vi "R vs T measurement.vi"() -> ()   [LabVIEW 2017]
uses:
  <vilib>/Utility/file.llb/Read Delimited Spreadsheet (DBL).vi
  <vilib>/Utility/file.llb/Write Delimited Spreadsheet (DBL).vi
  <instrlib>/Lake Shore 336/Lake Shore 336.lvlib
panel:
  in  "Tab Control":enum32{"Controlls", "Graphs"}(tab)
  in  "Source Meter address":refnum<visa-resource-name>="GPIB1::29::INSTR"
  out "Measured Resistance (Ohms)":dbl format="%#_6p"
  in  "Resistance Range Lower Limit (2 Ohm)":dbl=2.0 format="%#_6p"
  in  "Resistance Range Upper Limit (2E+8 Ohm)":dbl=200000000.0 format="%#_6p"
  in  "Resistance NPLC (0.1)":dbl=0.1
  in  "Resistance Range (2 Ohm)":dbl=2.0
  in  "Resistance Auto Range (T: Enable)":bool=TRUE
  in  "file to save data (dialog if empty)":path
  in  "Temperature controller Addres":refnum<visa-resource-name>
  in  "Input (0:A)":u16(ring) items=["A", "B", "C", "D"]
  in  "Range (0:Off)":u16(ring) items=["Off", "Low (On)", "Medium", "High"]
  in  "Manual Output (0.00 %)":dbl format="%.2f"
  in  "Setpoint (0.00000)":dbl format="%.5f"
  in  "Enable Setpoint (F:Off)":bool
  out "Measured Resistance (K)":dbl format="%.6p"
  in  "Ramp Rate (0.0)":dbl format="%.1f"
  in  "Setpoint Ramping \nEnable (F: Off)":bool
  in  "Output's Control Loop (1:1)":u16(ring)=1 items=["1"=1, "2"=2]
  in  "Rate (D) (0.0 %)":dbl format="%.1f"
  in  "Reset (I) (20.0)":dbl=20.0 format="%.1f"
  in  "Gain (P) (50.0)":dbl=50.0 format="%.1f"
  in  "Mode (0:Off)":u16(ring) items=["Off", "Closed Loop PID", "Zone", "Open Loop"]
  in  "Max User Current (2.000)":dbl=2.0 format="%.3f"
  in  "Max Current (0:User Specified)":u16(ring) items=["User Specified", "0.707 A", "1.0 A", "1.141 A", "2.0 A"]
  in  "Heater Out Display (1:Current)":u16(ring)=1 items=["Current"=1, "Power"=2]
  in  "Heater Resistance (1:25 Ohms)":u16(ring)=1 items=["25 Ohms"=1, "50 Ohms"=2]
  in  "Record Rate (ms)":u32=1000
  out "R T Graph":cluster{"all rows":dbl[], "all rows":dbl[]}(graph)
  in  "stop":bool
  in  "Error In":errorcluster
  # "Resistance vs Temperature Measurement"
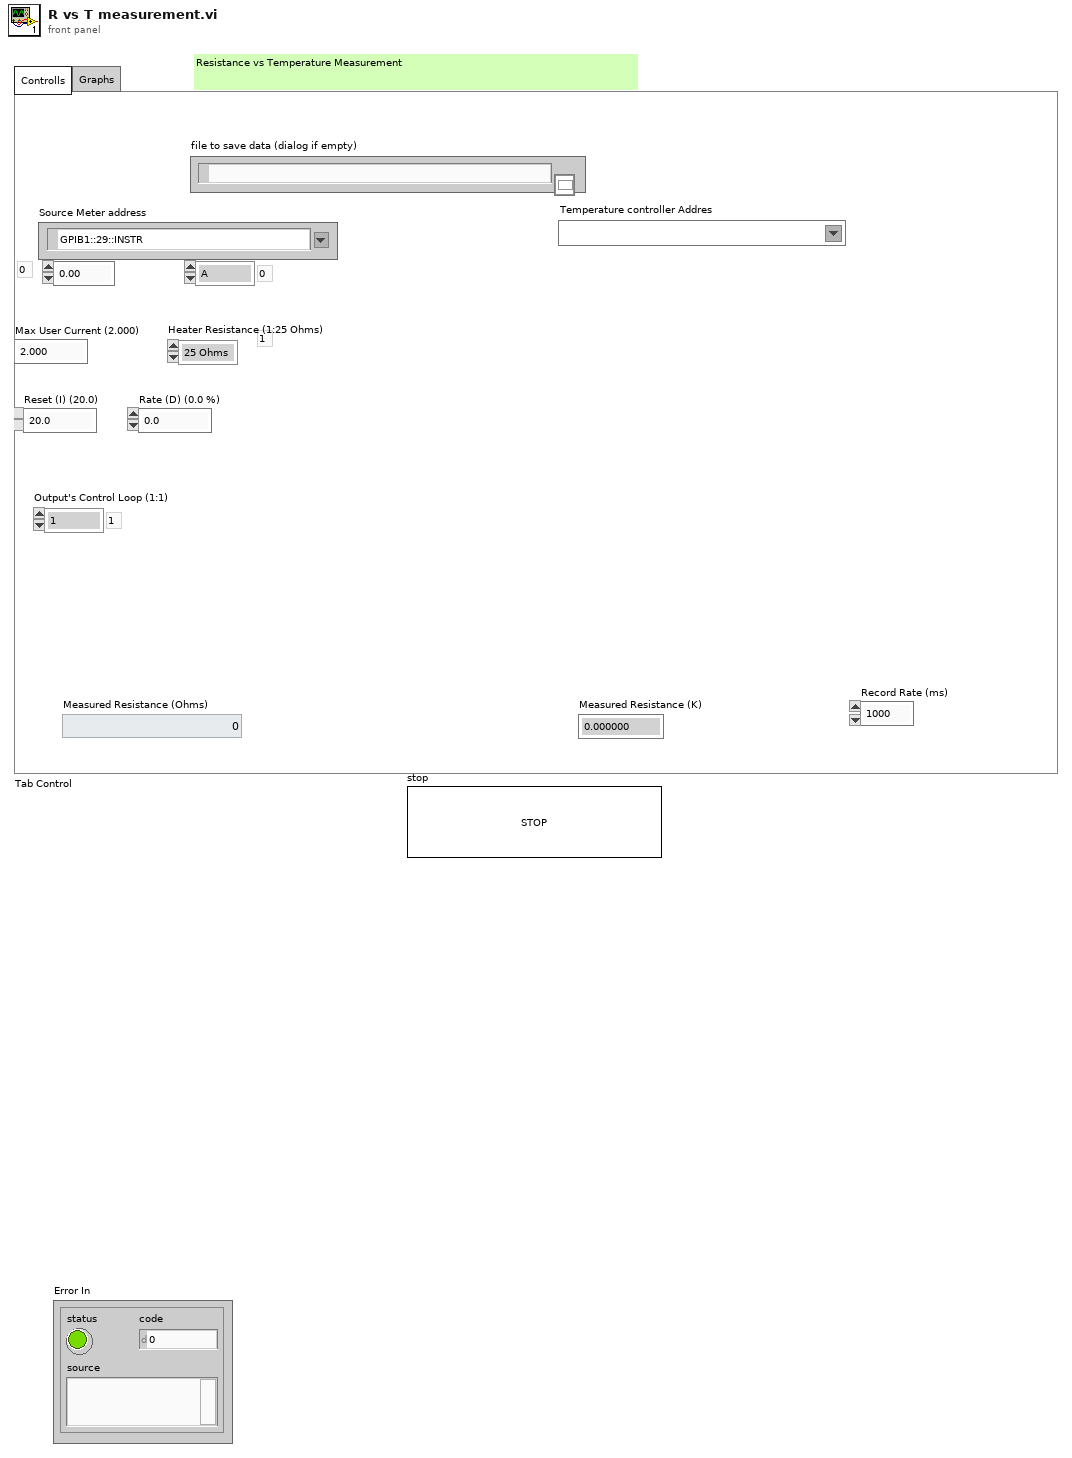
[diagram p1: front panel]
types:
  T1 = cluster{"Baud Rate":u32, "Parity":u16, "Data Bits":u16, "Stop Bits":u16, "Flow Control":u16}
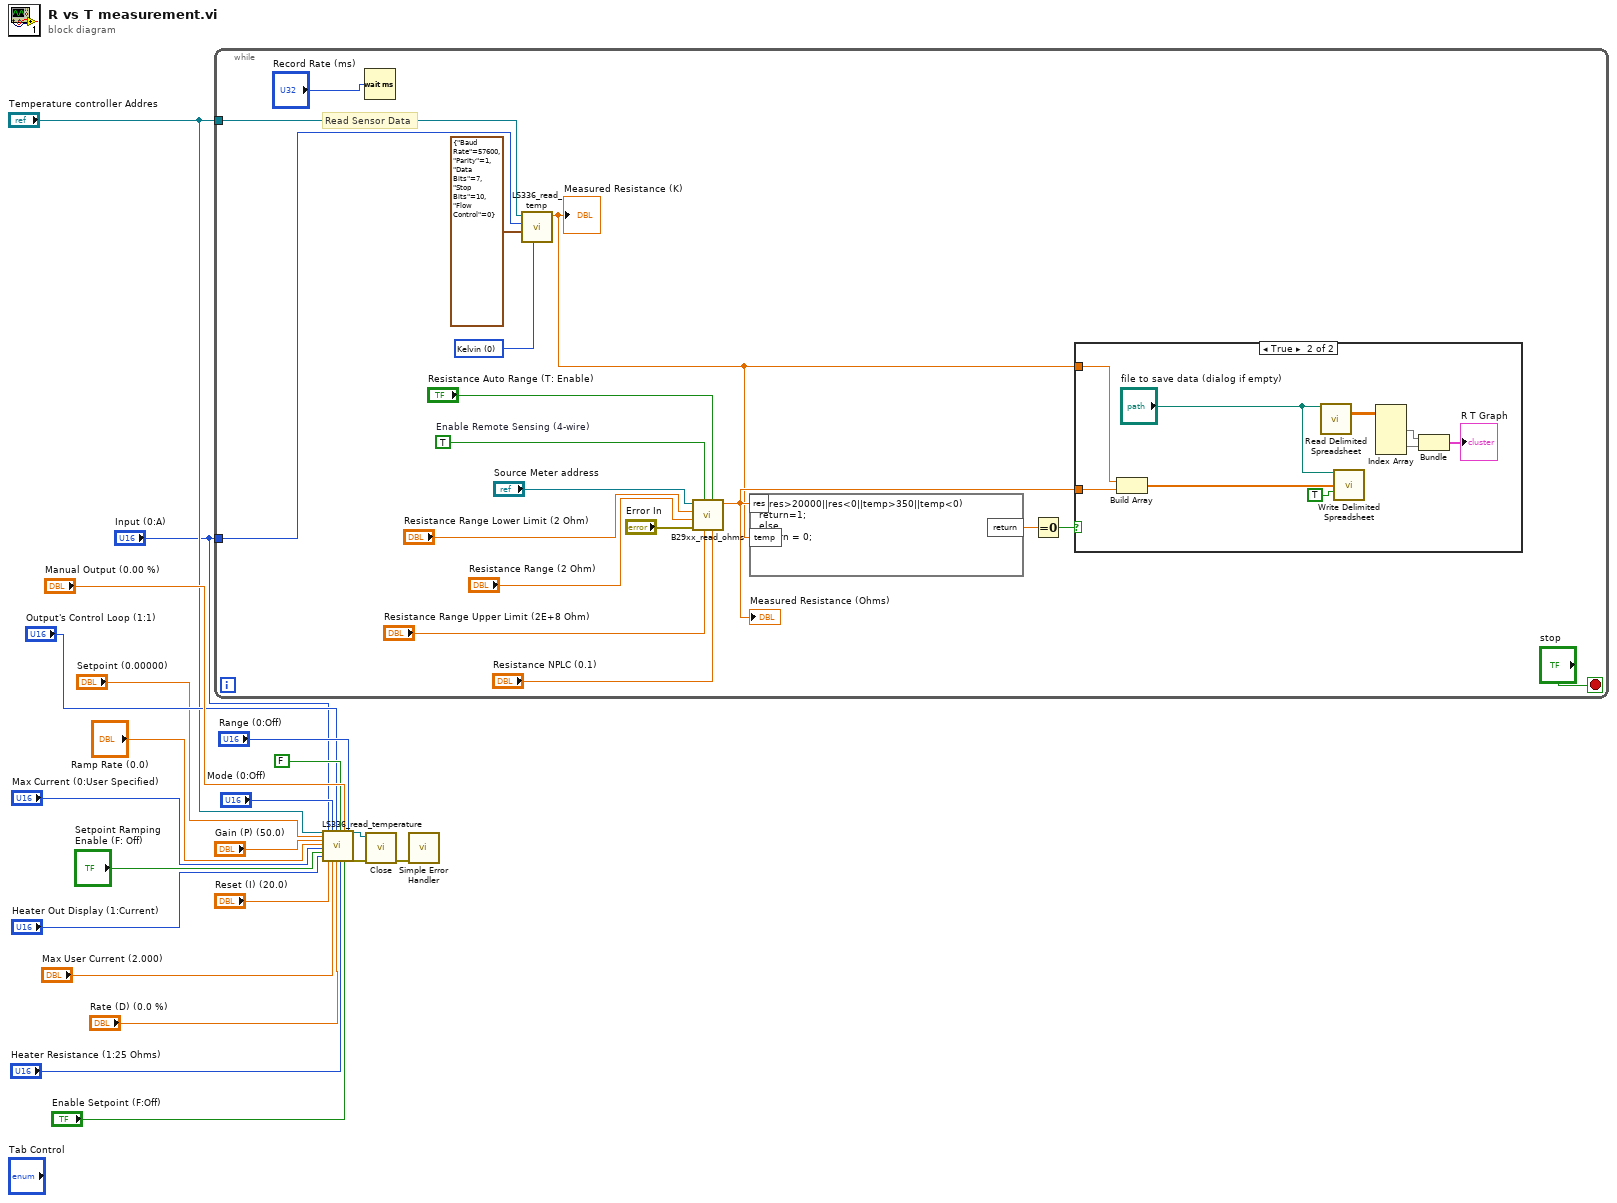
[diagram p0: block diagram]
diagram:
  n1 = while {
    tunnel: "Temperature controller Addres" -> [w23]
    tunnel: "Input (0:A)" -> [w22]
    stop <- "stop" stop-if-true
    w25 = u16 0 items=["Kelvin", "Celsius", "Sensor Units"] ("Data Source (0:Kelvin)")
    w37 = TRUE  # Enable Remote Sensing (4-wire)
    # "Read Sensor Data"
    n2 = Wait (ms)(milliseconds to wait="Record Rate (ms)") -> ()  [unwired: 1 out]
    n3 = call "LS336_read_temp.vi"("Data Source (0:Kelvin)"=w25, "Serial Configuration"=T1 {"Baud Rate"=57600, "Parity"=1, "Data Bits"=7, "Stop Bits"=10, "Flow Control"=0}, "Input (0:A)"=w22, "VISA Refnum in"=w23) -> ("Sensor Data"=w24:dbl)  [unwired: 7 in]
    "Measured Resistance (K)" <- w24
    n4 = call "B29xx_read_ohms.vi"("Resistance NPLC (0.1)"="Resistance NPLC (0.1)", "Resistance Auto Range (T: Enable)"="Resistance Auto Range (T: Enable)", "Resistance Range Upper Limit (2E+8 Ohm)"="Resistance Range Upper Limit (2E+8 Ohm)", "Enable Remote Sensing (4-wire)"=w37, "error in (no error)"="Error In", "Resistance Range (2 Ohm)"="Resistance Range (2 Ohm)", "Resistance Range Lower Limit (2 Ohm)"="Resistance Range Lower Limit (2 Ohm)", "VISA Refnum in"="Source Meter address") -> ("Measurement Result"=w29:dbl)  [unwired: 2 in, 1 out]
    "Measured Resistance (Ohms)" <- w29
    n5 = formula code="if(res>20000||res<0||temp>350||temp<0)\nreturn=1;\nelse \nreturn = 0;"("res"=w29, "temp"=w24) -> ("return"=w31:dbl)
    n6 = Equal To 0?(x=w31) -> (x = 0?=w30:bool)
    n7 = case shown="True" w30 {
      tunnel: w29 -> [_ w46]
      tunnel: w24 -> [_ w40]
      frame False {
      }
      frame True {
        n8 = Build Array(w40, w46) -> (w47:dbl[])
        n9 = call-poly <vilib>:"Read Delimited Spreadsheet.vi"("file path (dialog if empty)"="file to save data (dialog if empty)") -> ("all rows"=w42:dbl[][])  [unwired: 9 in, 5 out]
        n10 = call-poly <vilib>:"Write Delimited Spreadsheet.vi"("file path (dialog if empty)"="file to save data (dialog if empty)", "1D data"=w47, "append to file? (new file:F)"=TRUE) -> ()  [unwired: 11 in, 2 out]
        n11 = Index Array(array=w42) -> (element #1=w43:dbl[], element #2=w44:dbl[])  [unwired: 4 in]
        n12 = Bundle("all rows"=w43, "all rows"=w44) -> (→"R T Graph":cluster{"all rows":dbl[], "all rows":dbl[]})  [unwired: 1 in]
      }
    }
  }
  n13 = call "LS336_read_temperature.vi"("VISA Refnum in"="Temperature controller Addres", "Setpoint (0.00000)"="Setpoint (0.00000)", "Gain (P) (50.0)"="Gain (P) (50.0)", "Ramp Rate (0.0)"="Ramp Rate (0.0)", "Max Current (0:User Specified)"="Max Current (0:User Specified)", "Setpoint Ramping \nEnable (F: Off)"="Setpoint Ramping \nEnable (F: Off)", "Heater Out Display (1:Current)"="Heater Out Display (1:Current)", "Input (0:None)"="Input (0:A)", "Reset (I) (20.0)"="Reset (I) (20.0)", "Mode (0:Off)"="Mode (0:Off)", "Max User Current (2.000)"="Max User Current (2.000)", "Output's Control Loop (1:1)"="Output's Control Loop (1:1)", "Rate (D) (0.0 %)"="Rate (D) (0.0 %)", "Power Up Enable (F: Off)"=FALSE, "Heater Resistance (1:25 Ohms)"="Heater Resistance (1:25 Ohms)", "Manual Output (0.00 %)"="Manual Output (0.00 %)", "Enable Setpoint (F:Off)"="Enable Setpoint (F:Off)", "Range (0:Off)"="Range (0:Off)") -> ("VISA Refnum out"=w20:refnum<visa-resource-name>, "error out"=w21:errorcluster)  [unwired: 8 in]
  n14 = call <instrlib>:"Close.vi"("error in (no error)"=w21, "VISA resource name"=w20) -> ("error out"=w7:errorcluster)  [unwired: 9 in]
  n15 = call <vilib>:"Simple Error Handler.vi"("error in (no error)"=w7) -> ()  [unwired: 4 in, 5 out]
